vi "Write period.vi"(8 "error in (no error)":errorcluster, 10 "period":u16=4000, 11 "rqcBob in":refnum<class "rqcBob.lvclass">) -> (0 "error out":errorcluster, 3 "rqcBob out":refnum<class "rqcBob.lvclass">)   [LabVIEW 2019, in "rqcBob.lvclass"]
uses:
  rqcBob.lvclass
  Custom Controls/rqcBob Main FPGA interface.ctl
  rqcBob.lvclass/rqcBob.ctl
  <vilib>/Utility/error.llb/Error Cluster From Error Code.vi
  <vilib>/rvi/errors/niLvFpgaAdjustHostInterfaceError.vi
  <vilib>/rvi/interface/nirviReadWriteControl/nirviReadWriteControl.xnode
  NiFpgaLv.dll
  <vilib>/rvi/interface/Simulation/niFpgaSimulationCallBeginRW.vi
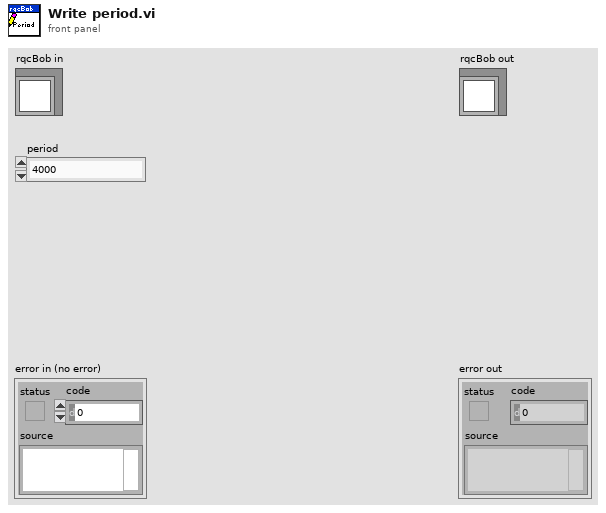
[diagram p1: front panel]
types:
  T1 = typedef "rqcBob.lvclass/rqcBob Main FPGA interface.ctl" = refnum<k20>
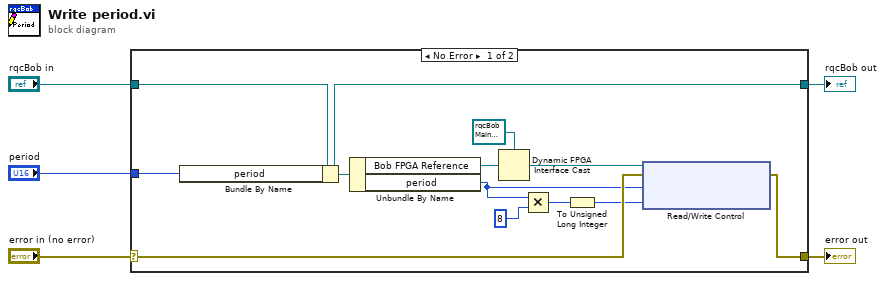
[diagram p0: block diagram]
diagram:
  n1 = case shown="No Error" "error in (no error)" {
    selector: "error in (no error)" -> [w11 w18]
    tunnel: [w10 w18] -> w4
    tunnel: [w15 w19] -> w2
    tunnel: "rqcBob in" -> [w17 w19]
    tunnel: "period" -> [w16 _]
    frame No Error {
      n2 = Bundle By Name(cluster=w17, "period"=w16) -> (w15:refnum<class "rqcBob.lvclass">)
      n3 = Unbundle By Name(w15) -> ("Bob FPGA Reference"=w14:refnum<k20>, "period"=w7:u16)
      n4 = Dynamic FPGA Interface Cast(Session In=T1 refnum ("Bob main FPGA interface"), Type=w14) -> (Session Out=w12:T1)
      n5 = Multiply(x=w7, y=u16 8) -> (x*y=w8:u16)
      n6 = To Unsigned Long Integer(number=w8) -> (unsigned 32bit integer=w6:u32)
      n7 = xnode "Read/Write Control"("FPGA VI Reference In"=w12, "error in"=w11, "train.period"=w7, "PD.max meas length"=w6) -> ("error out"=w10:errorcluster)  [unwired: 1 out]
    }
    frame Error {
    }
  }
  "error out" <- w4
  "rqcBob out" <- w2
